vi "Msg.vi"(7 "jettl in":refnum<class "jettl.lvclass">, 11 "Last Ack Event Msg Strategy in":refnum<class "Last Ack Event Msg Strategy.lvclass">) -> (5 "jettl out":refnum<class "jettl.lvclass">)   [LabVIEW 2021, in "jettl.lvlib" / "jettl Msg Last Ack Event.lvlib" / "Last Ack Event Msg Strategy.lvclass"]
uses:
  Last Ack Event Msg Strategy.lvclass
  Last Ack Event Msg Strategy.lvclass/Last Ack Event Msg Strategy.ctl
  Last Ack Event/Last Ack Event.lvclass
  jettl/jettl.lvclass
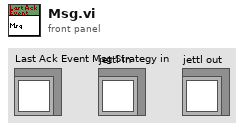
[diagram p1: front panel]
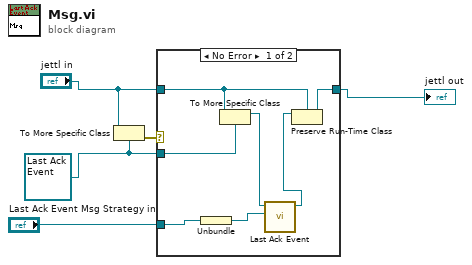
[diagram p0: block diagram]
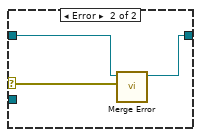
[diagram p2: hidden frame]
diagram:
  w3 = refnum<class "Last Ack Event.lvclass"> refnum ("Event Last Ack.lvlib:Event Last Ack.lvclass")
  n1 = To More Specific Class(target class=w3, reference="jettl in") -> (error out=w5:errorcluster)  [unwired: 1 in, 1 out]
  n2 = case shown="No Error" w5 {
    selector: w5 -> [_ w15]
    tunnel: [w10 w13] -> w1
    tunnel: "jettl in" -> [w11 w14]
    tunnel: w3 -> [w12 _]
    tunnel: "Last Ack Event Msg Strategy in" -> [w7 _]
    frame No Error {
      n3 = Unbundle(w7) -> (w6:refnum<class "Event jettl.lvclass">)
      n4 = To More Specific Class(target class=w12, reference=w11) -> (specific class reference=w9:refnum<class "Last Ack Event.lvclass">)  [unwired: 1 in, 1 out]
      n5 = call-dynamic "Last Ack Event.vi"("Event jettl"=w6, "Last Ack Event in"=w9) -> ("Last Ack Event out"=w8:refnum<class "Last Ack Event.lvclass">)  [unwired: 9 in]
      n6 = Preserve Run-Time Class(object in=w8, 2:w11) -> (object out=w10:refnum<class "jettl.lvclass">)  [unwired: 1 in, 1 out]
    }
    frame Error {
      n7 = call-dynamic "Merge Error.vi"("Error"=w15, "Merge Error in"=w14) -> ("Merge Error out"=w13:refnum<class "jettl.lvclass">)  [unwired: 9 in]
    }
  }
  "jettl out" <- w1
